vi "ConvertToADCReading.vi"(2 "Temperature / C":dbl=25.0 format="%#_13g", 3 "Input arm settings":T1={"Vref"=1.0, "Rgain"=100000.0, "Rset"=10000.0, "Rseries"=1000.0, "Input polarity?"=FALSE}) -> (0 "I":dbl=9.999956835536101e-05, 1 "Reading / V":dbl=1.726578555962758e-05)   [LabVIEW 2015]
uses:
  <vilib>/imath/engines/lvmath2/RunTimeEngine/ArithmeticOperatorToken/NIMS_ArithmeticOperator_power(S).vi
  <instcachedir>/0/NIMS_ArithmeticOperator_power(S)_DFB67823F1414E5097C86E39787D8CA8.lvgen/NIMS_ArithmeticOperator_power(S)_DFB67823F1414E5097C86E39787D8CA8_009.vi
  <vilib>/imath/engines/lvmath2/RunTimeEngine/ErrorHandling/NIMS_Create Error From Enums.vi
  <vilib>/imath/engines/lvmath2/RunTimeEngine/NodeEndStatement/NIMS_NodeEndStatement_Output.vi
  <instcachedir>/0/NIMS_NodeEndStatement_Output_53EC0D466D134D7ABD903AC30B43404B.lvgen/NIMS_NodeEndStatement_Output_53EC0D466D134D7ABD903AC30B43404B_009.vi
  <vilib>/imath/engines/lvmath2/RunTimeEngine/ErrorHandling/NIMS_Finalize Error.vi
panel:
  out "Rtherm":cdb
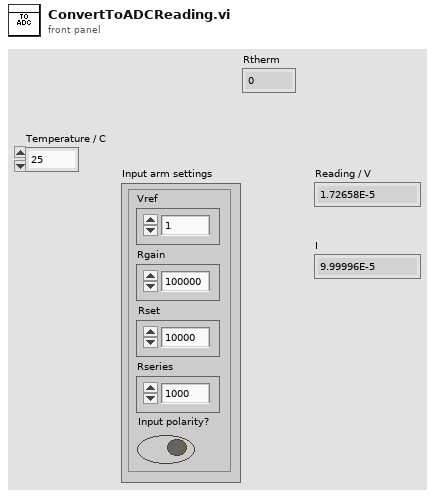
[diagram p1: front panel]
types:
  T1 = cluster{"Vref":dbl, "Rgain":dbl, "Rset":dbl, "Rseries":dbl, "Input polarity?":bool}
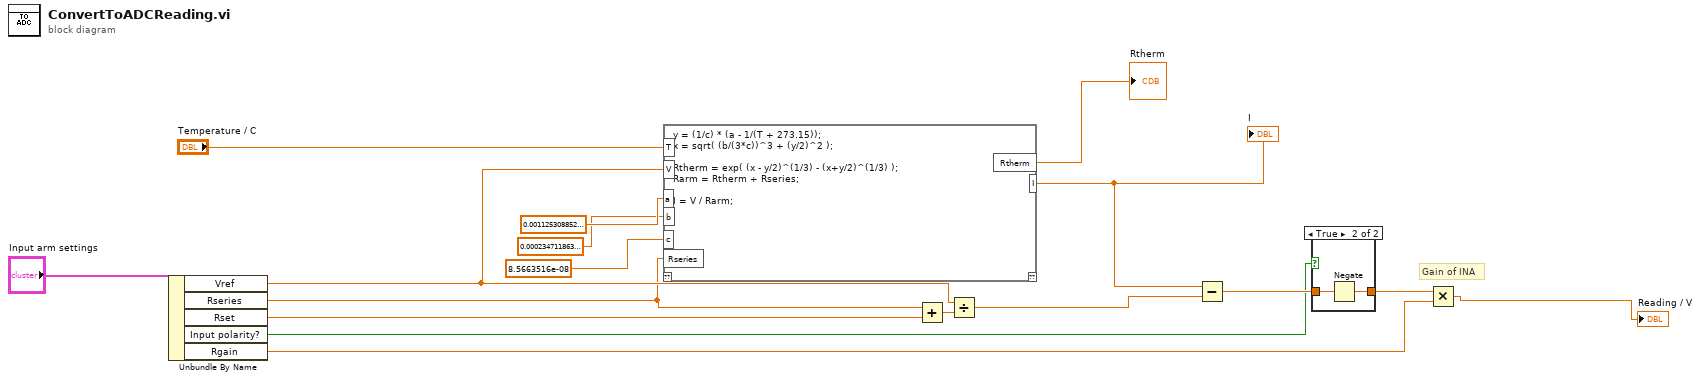
[diagram p0: block diagram]
diagram:
  # "Gain of INA"
  n1 = Unbundle By Name("Input arm settings") -> ("Vref"=w3:dbl, "Rseries"=w1:dbl, "Rset"=w2:dbl, "Input polarity?"=w4:bool, "Rgain"=w5:dbl)
  n2 = mathscript code="y = (1/c) * (a - 1/(T + 273.15));\nx = sqrt( (b/(3*c))^3 + (y/2)^2 );\n\nRtherm = exp( (x - y/2)^(1/3) - (x+y/2)^(1/3) );\nRarm = Rtherm + Rseries;\n\nI = V / Rarm;"("T"="Temperature / C", "V"=w3, "a"=0.001125308852122, "b"=0.000234711863267, "c"=8.5663516e-08, "Rseries"=w1) -> ("I"=w15:cdb, "Rtherm"=→"Rtherm":cdb)  [unwired: 1 in, 1 out]
  "I" <- w15
  n3 = Add(x=w1, y=w2) -> (x+y=w10:dbl)
  n4 = Divide(x=w3, y=w10) -> (x/y=w9:dbl)
  n5 = Subtract(x=w15, y=w9) -> (x-y=w17:cdb)
  n6 = case shown="True" w4 {
    tunnel: w17 -> [w18 w20]
    tunnel: [w18 w19] -> w16
    frame False {
    }
    frame True {
      n7 = Negate(x=w20) -> (-x=w19:cdb)
    }
  }
  n8 = Multiply(x=w16, y=w5) -> (x*y=→"Reading / V":cdb)
